vi "GOOP_SetCustomClassTemplates.vi"(10 "ClassType":string, 11 "CustomTemplates":path[](array[path])) -> ()   [LabVIEW 2020]
uses:
  <vilib>/Utility/config.llb/Write Key (Path).vi
  <vilib>/Utility/config.llb/NI_LVConfig.lvlib
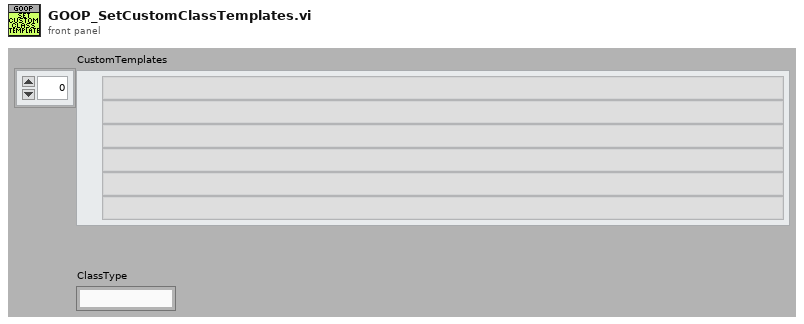
[diagram p1: front panel]
types:
  T1 = typedef "NI_LVConfig.lvlib/Config Data RefNum.ctl" = refnum<k1>
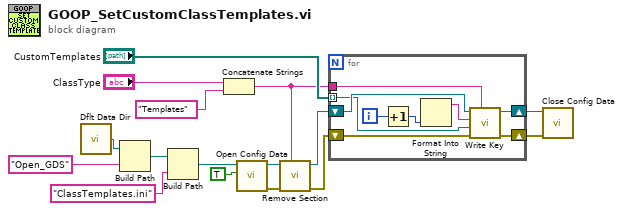
[diagram p0: block diagram]
diagram:
  n1 = call <vilib>:"Dflt Data Dir.vi"() -> ("App:Default Data Directory"=w16:path)
  n2 = Build Path(base path=w16, name or relative path="Open_GDS") -> (appended path=w14:path)
  n3 = Build Path(base path=w14, name or relative path="ClassTemplates.ini") -> (appended path=w9:path)
  n4 = Concatenate Strings("ClassType", "Templates" ("string")) -> (w1:string)
  n5 = call <vilib>:"Open Config Data.vi"("create file if necessary (T)"=TRUE, "configuration file path"=w9) -> ("error out"=w7:errorcluster, "refnum"=w8:T1)  [unwired: 7 in, 1 out]
  n6 = call <vilib>:"Remove Section.vi"("section"=w1, "error in (no error)"=w7, "refnum"=w8) -> ("error out"=w4:errorcluster, "refnum out"=w6:T1)  [unwired: 6 in, 1 out]
  n7 = for {
    shift-right: [w22] -> w3
    shift-left: w4 -> [w23]
    shift-right: [w24] -> w5
    shift-left: w6 -> [w25]
    tunnel: "CustomTemplates" -> [w21] mode=indexing
    tunnel: w1 -> [w17]
    i -> [w19]
    n8 = Increment(x=w19) -> (x+1=w20:i32)
    n9 = Format Into String(w20) -> (resulting string=w18:string)  [unwired: 3 in, 1 out]
    n10 = call-poly <vilib>:"Write Key.vi"("section"=w17, "error in (no error)"=w23, "value"=w21, "key"=w18, "refnum"=w25) -> ("error out"=w22:errorcluster, "refnum out"=w24:T1)  [unwired: 4 in, 1 out]
  }
  n11 = call <vilib>:"Close Config Data.vi"("error in (no error)"=w3, "refnum"=w5) -> ()  [unwired: 8 in, 2 out]
